vi "1WIRE_RESET_9402.vi"(8 "error in":errorcluster) -> (0 "error out":errorcluster, 1 "0 = Device Present / 1=no":bool)   [LabVIEW 2012]
doc: "This VI is created by Vincent Claes for FPDA-1 more information on http://pwo.fpga.be\n\nvincent.claes@xios.be\nclaesvincent@gmail.com\n\nhttp://www.linkedin.com/in/vincentclaes"
uses:
  <vilib>/rvi/Emulation/niFpgaSctlEmulationGetInTimedLoop.vi
  <vilib>/rvi/Emulation/niFpgaSctlEmulationGlobalWrite.vi
  <vilib>/rvi/eio/common/nirviEmuTemplateMethod_errors.vi
  <vilib>/eio/EIOMethodNode/EIOMethodNode.xnode
  <vilib>/eio/EIONode/EIONode.xnode
panel:
  out "x-y 5":u32
  out "x-y 4":u32
  out "x-y 3":u32
  out "x-y 2":u32
  out "x-y":u32
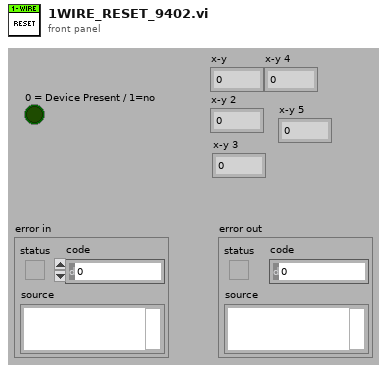
[diagram p1: front panel]
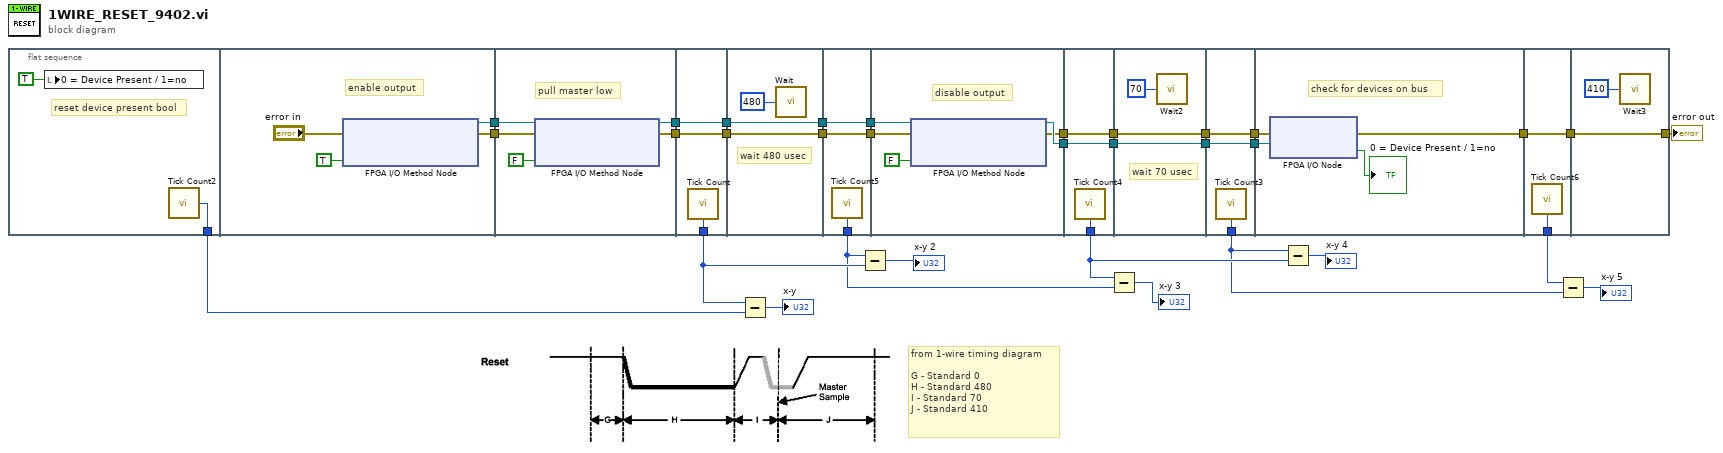
[diagram p0: block diagram]
diagram:
  # "from 1-wire timing diagram\n\nG - Standard 0\nH - Standard 480\nI - Standard 70\nJ - Standard 410"
  n1 = flat-sequence {
    tunnel: [w33] -> w25
    tunnel: [w37] -> w32
    tunnel: [w36] -> w31
    tunnel: w32 -> [w43]
    tunnel: w31 -> [w42]
    tunnel: [w41] -> w29
    tunnel: [w40] -> w27
    tunnel: w29 -> [w46]
    tunnel: [w46] -> w28
    tunnel: w27 -> [w45]
    tunnel: [w45] -> w26
    tunnel: [w44] -> w8
    tunnel: [w48] -> w24
    tunnel: w28 -> [w48]
    tunnel: w26 -> [w47]
    tunnel: [w47] -> w22
    tunnel: w24 -> [w52]
    tunnel: [w52] -> w23
    tunnel: w22 -> [w51]
    tunnel: [w51] -> w21
    tunnel: [w50] -> w6
    tunnel: [w56] -> w20
    tunnel: [w55] -> w18
    tunnel: w23 -> [w54]
    tunnel: w21 -> [w53]
    tunnel: w20 -> [w60]
    tunnel: [w60] -> w19
    tunnel: w18 -> [w59]
    tunnel: [w59] -> w17
    tunnel: [w58] -> w12
    tunnel: [w62] -> w16
    tunnel: w19 -> [w62]
    tunnel: w17 -> [w61]
    tunnel: [w61] -> w14
    tunnel: w16 -> [w66]
    tunnel: [w66] -> w15
    tunnel: w14 -> [w65]
    tunnel: [w65] -> w13
    tunnel: [w64] -> w1
    tunnel: w15 -> [w69]
    tunnel: w13 -> [w68]
    tunnel: [w67] -> w10
    tunnel: w10 -> [w72]
    tunnel: [w72] -> w9
    tunnel: [w71] -> w2
    tunnel: w9 -> [w73]
    tunnel: [w73] -> w30
    frame #0 {
      # "reset device present bool"
      n2 = local write "0 = Device Present / 1=no"(TRUE ("0 = Device Present / 1=no")) -> ()
      n3 = call "Tick Count2"() -> ("Tick Count(uSec)"=w33:u32)
    }
    frame #1 {
      # "enable output"
      n4 = xnode "FPGA I/O Method Node"("error in"="error in", "Enable"=TRUE ("Data")) -> ("error out"=w36:errorcluster, "FPGA I/O Out"=w37:refnum<k21>)  [unwired: 1 in]
    }
    frame #2 {
      # "pull master low"
      n5 = xnode "FPGA I/O Method Node"("error in"=w42, "FPGA I/O In"=w43, "Data"=FALSE ("FX2_IO1_J1_0")) -> ("error out"=w40:errorcluster, "FPGA I/O Out"=w41:refnum<k21>)
    }
    frame #3 {
      n6 = call "Tick Count"() -> ("Tick Count(uSec)"=w44:u32)
    }
    frame #4 {
      # "wait 480 usec"
      n7 = call "Wait"("Count(uSec)"=u32 480) -> ()  [unwired: 1 out]
    }
    frame #5 {
      n8 = call "Tick Count5"() -> ("Tick Count(uSec)"=w50:u32)
    }
    frame #6 {
      # "disable output"
      n9 = xnode "FPGA I/O Method Node"("error in"=w53, "FPGA I/O In"=w54, "Enable"=FALSE ("Data")) -> ("error out"=w55:errorcluster, "FPGA I/O Out"=w56:refnum<k21>)
    }
    frame #7 {
      n10 = call "Tick Count4"() -> ("Tick Count(uSec)"=w58:u32)
    }
    frame #8 {
      # "wait 70 usec"
      n11 = call "Wait2"("Count(uSec)"=u32 70) -> ()  [unwired: 1 out]
    }
    frame #9 {
      n12 = call "Tick Count3"() -> ("Tick Count(uSec)"=w64:u32)
    }
    frame #10 {
      # "check for devices on bus"
      n13 = xnode "FPGA I/O Node"("error in"=w68, "FPGA I/O In"=w69) -> ("error out"=w67:errorcluster, "I/O Item"=→"0 = Device Present / 1=no":bool)  [unwired: 1 out]
    }
    frame #11 {
      n14 = call "Tick Count6"() -> ("Tick Count(uSec)"=w71:u32)
    }
    frame #12 {
      n15 = call "Wait3"("Count(uSec)"=u32 410) -> ()  [unwired: 1 out]
    }
  }
  n16 = Subtract(x=w8, y=w25) -> (x-y=→"x-y":u32)
  n17 = Subtract(x=w6, y=w8) -> (x-y=→"x-y 2":u32)
  n18 = Subtract(x=w12, y=w6) -> (x-y=→"x-y 3":u32)
  n19 = Subtract(x=w1, y=w12) -> (x-y=→"x-y 4":u32)
  n20 = Subtract(x=w2, y=w1) -> (x-y=→"x-y 5":u32)
  "error out" <- w30
